vi "GetProperties.vi"(8 "error in":errorcluster, 11 "CompoundArithmetic in":refnum<class "CompoundArithmetic.lvclass">) -> (0 "error out":errorcluster, 3 "CompoundArithmetic out":refnum<class "CompoundArithmetic.lvclass">)   [LabVIEW 2014, in "CompoundArithmetic.lvclass"]
uses:
  CompoundArithmetic.lvclass
  CompoundArithmetic.lvclass/CompoundArithmetic.ctl
  GrowableFunction/GrowableFunction.lvclass
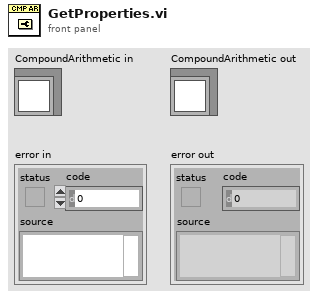
[diagram p1: front panel]
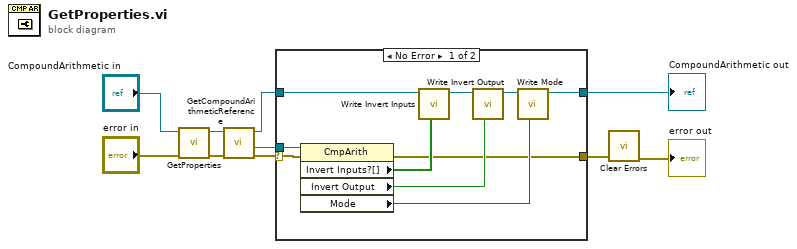
[diagram p0: block diagram]
diagram:
  n1 = call-parent "GetProperties.vi"("error in"="error in", "GObject in"="CompoundArithmetic in") -> ("error out"=w1:errorcluster, "GObject out"=w3:refnum<class "CompoundArithmetic.lvclass">)  [unwired: 8 in]
  n2 = call "GetCompoundArithmeticReference.vi"("error in"=w1, "NamedBundler in"=w3) -> ("error out"=w10:errorcluster, "reference out"=w9:refnum<vi>, "NamedBundler out"=w8:refnum<class "CompoundArithmetic.lvclass">)  [unwired: 7 in]
  n3 = case shown="No Error" w10 {
    selector: w10 -> [w19 w22]
    tunnel: w9 -> [w20 _]
    tunnel: w8 -> [w13 w21]
    tunnel: [w12 w21] -> w7
    tunnel: [w11 w22] -> w6
    frame No Error {
      n4 = property class="CmpArith"(reference=w20, error in=w19) -> (error out=w11:errorcluster, "Invert Inputs?[]"=w16:bool[], "Invert Output"=w17:bool, "Mode"=w18:u32)  [unwired: 1 out]
      n5 = call "Write Invert Inputs.vi"("Invert Inputs"=w16, "CompoundArithmetic in"=w13) -> ("CompoundArithmetic out"=w15:refnum<class "CompoundArithmetic.lvclass">)  [unwired: 7 in]
      n6 = call "Write Invert Output.vi"("Invert Output"=w17, "CompoundArithmetic in"=w15) -> ("CompoundArithmetic out"=w14:refnum<class "CompoundArithmetic.lvclass">)  [unwired: 7 in]
      n7 = call "Write Mode.vi"("Mode"=w18, "CompoundArithmetic in"=w14) -> ("CompoundArithmetic out"=w12:refnum<class "CompoundArithmetic.lvclass">)  [unwired: 7 in]
    }
    frame Error {
    }
  }
  "CompoundArithmetic out" <- w7
  n8 = call <vilib>:"Clear Errors.vi"("error in (no error)"=w6) -> ("error out"=→"error out":errorcluster)  [unwired: 5 in, 1 out]
